vi "analog signal_out.vi"(7 "stop":bool, 9 "amplitude":dbl=1.0 format="%0.2p", 10 "frequency":dbl=10.0 format="%0.2p") -> (3 "signal out":waveform(dbl))   [LabVIEW 2018]
uses:
  <vilib>/measure/NI_MABase.lvlib
panel:
  out "Waveform Graph":waveform(dbl)(graph)
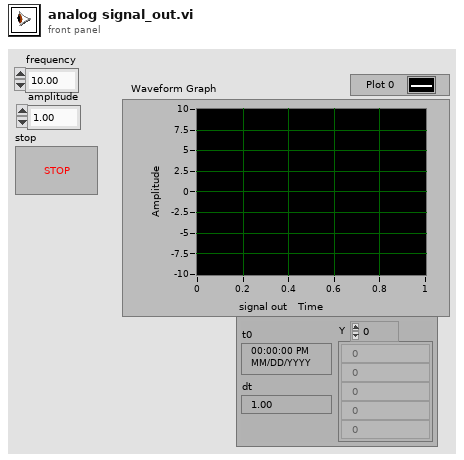
[diagram p1: front panel]
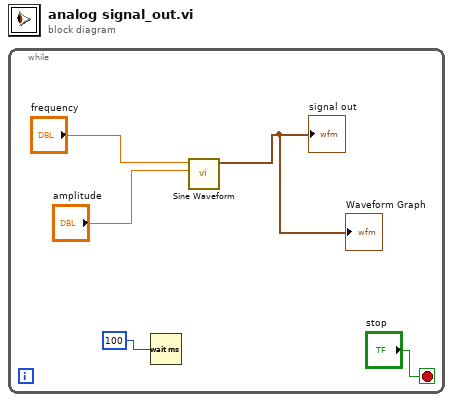
[diagram p0: block diagram]
diagram:
  n1 = while {
    stop <- "stop" stop-if-true
    n2 = Wait (ms)(milliseconds to wait=u32 100 ("millisecond timer value")) -> ()  [unwired: 1 out]
    n3 = call <vilib>:"Sine Waveform.vi"("amplitude"="amplitude", "frequency"="frequency") -> ("signal out"=→"Waveform Graph" →"signal out":waveform(dbl))  [unwired: 8 in, 1 out]
  }
